vi "GetAvPowerN1911a.vi"(6 "error in (no error)":errorcluster, 7 "NreadingsFromPwrMeter":i32=30 min=1 max=1000 step=1, 8 "IntervalBetweenReadings (mS)":i32=10 min=1 max=1000 step=1) -> (0 "Error out":errorcluster, 1 "VI dBSSD Power (dB)":dbl format="%#.10f", 2 "Computed LinMean Power (dBm)":dbl format="%#.10f", 3 "VI dBMean Power (dBm)":dbl format="%#.10f")   [LabVIEW 2009]
doc: "Reads the power from the N1911A power meter."
uses:
  <vilib>/Analysis/NI_AALBase.lvlib
panel:
  out "PwrAveragingLoopCount":i32
  in  "HistogramIntervals":i32=50 min=1 max=1000 step=1
  out "dB Readings Histogram":T1(graph)
  # "Get and discard\n1 initial value.\nMust we do this?"
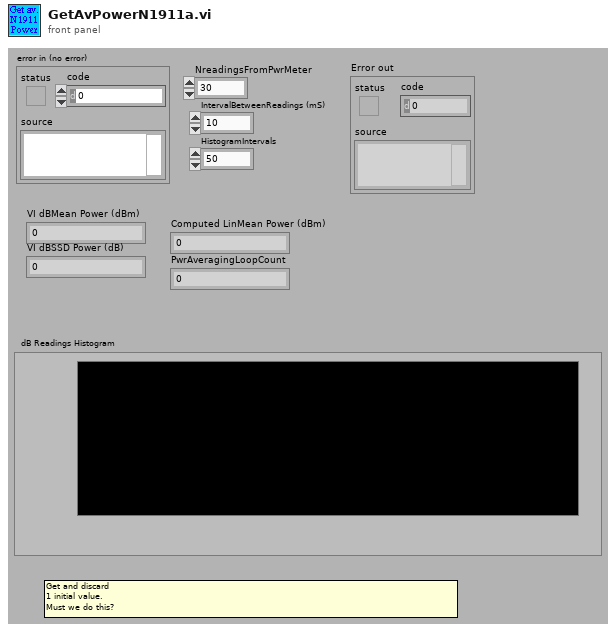
[diagram p1: front panel]
types:
  T1 = cluster{"X Values":dbl[], "Histogram: h(x)":i32[]}
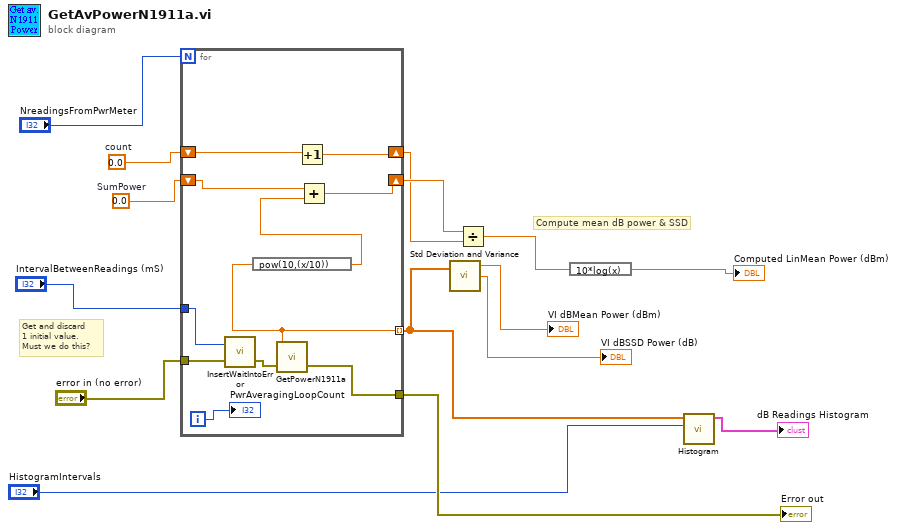
[diagram p0: block diagram]
diagram:
  w12 = 0.0  # count
  w15 = 0.0  # SumPower
  # "Get and discard\n1 initial value.\nMust we do this?"
  # "Compute mean dB power & SSD"
  n1 = for {
    N: "NreadingsFromPwrMeter" -> [_]
    shift-right: [w25] -> w14
    shift-left: w15 -> [w26]
    tunnel: [w24] -> w4
    shift-right: [w22] -> w11
    shift-left: w12 -> [w23]
    tunnel: [w19] -> w3 mode=indexing
    tunnel: "IntervalBetweenReadings (mS)" -> [w20]
    tunnel: "error in (no error)" -> [w16]
    i -> [w17]
    n2 = call "InsertWaitIntoError.vi"("error in (no error)"=w16, "Wait (msecs)"=w20) -> ("error out"=w21:errorcluster)  [unwired: 1 in]
    n3 = call "GetPowerN1911a.vi"("error in (no error)"=w21) -> ("Error out"=w24:errorcluster, "Power returned (dBm)"=w19:dbl)  [unwired: 1 in]
    n4 = expression code="pow(10,(x/10))"(w19) -> (w18:dbl)
    n5 = Increment(x=w23) -> (x+1=w22:dbl)
    n6 = Add(x=w26, y=w18) -> (x+y=w25:dbl)
    "PwrAveragingLoopCount" <- w17
  }
  "Error out" <- w4
  n7 = call <vilib>:"Std Deviation and Variance.vi"("X"=w3) -> ("mean"=→"VI dBMean Power (dBm)":dbl, "standard deviation"=→"VI dBSSD Power (dB)":dbl)  [unwired: 1 in, 1 out]
  n8 = Divide(x=w14, y=w11) -> (x/y=w7:dbl)
  n9 = expression code="10*log(x)"(w7) -> (→"Computed LinMean Power (dBm)":dbl)
  n10 = call <vilib>:"Histogram.vi"("intervals"="HistogramIntervals", "X"=w3) -> ("Histogram Graph"=→"dB Readings Histogram":T1)  [unwired: 6 in, 3 out]
